vi "AudioTest.Plot, Normalize Freq Response Plot.vi"(6 "Average(F), Center_Min_Max(T)":bool, 8 "F End":dbl=20000.0, 9 "F Start":dbl=500.0, 11 "Data In":T1) -> (1 "Avg Level":T2 {"Status" items=["LOG", "PASS", "FAIL", "ERROR"]}, 3 "Data Out":T1)   [LabVIEW 2018]
uses:
  TypeDefs/AudioTest.Result Plot Data.ctl
  Common/Utils/Results/Result.Numeric.ctl
  Common/Utils/Results/Result.Limit Type.ctl
  Common/Utils/Results/Result.Measurement and Attribute Item Status.ctl
panel:
  in  "Limits In":T1[](array[typedef])
  out "XY Graph Out":cluster{"X":dbl[], dbl[]}(graph)
  out "XY Graph":cluster{"X":dbl[], "Y":dbl[]}(graph)
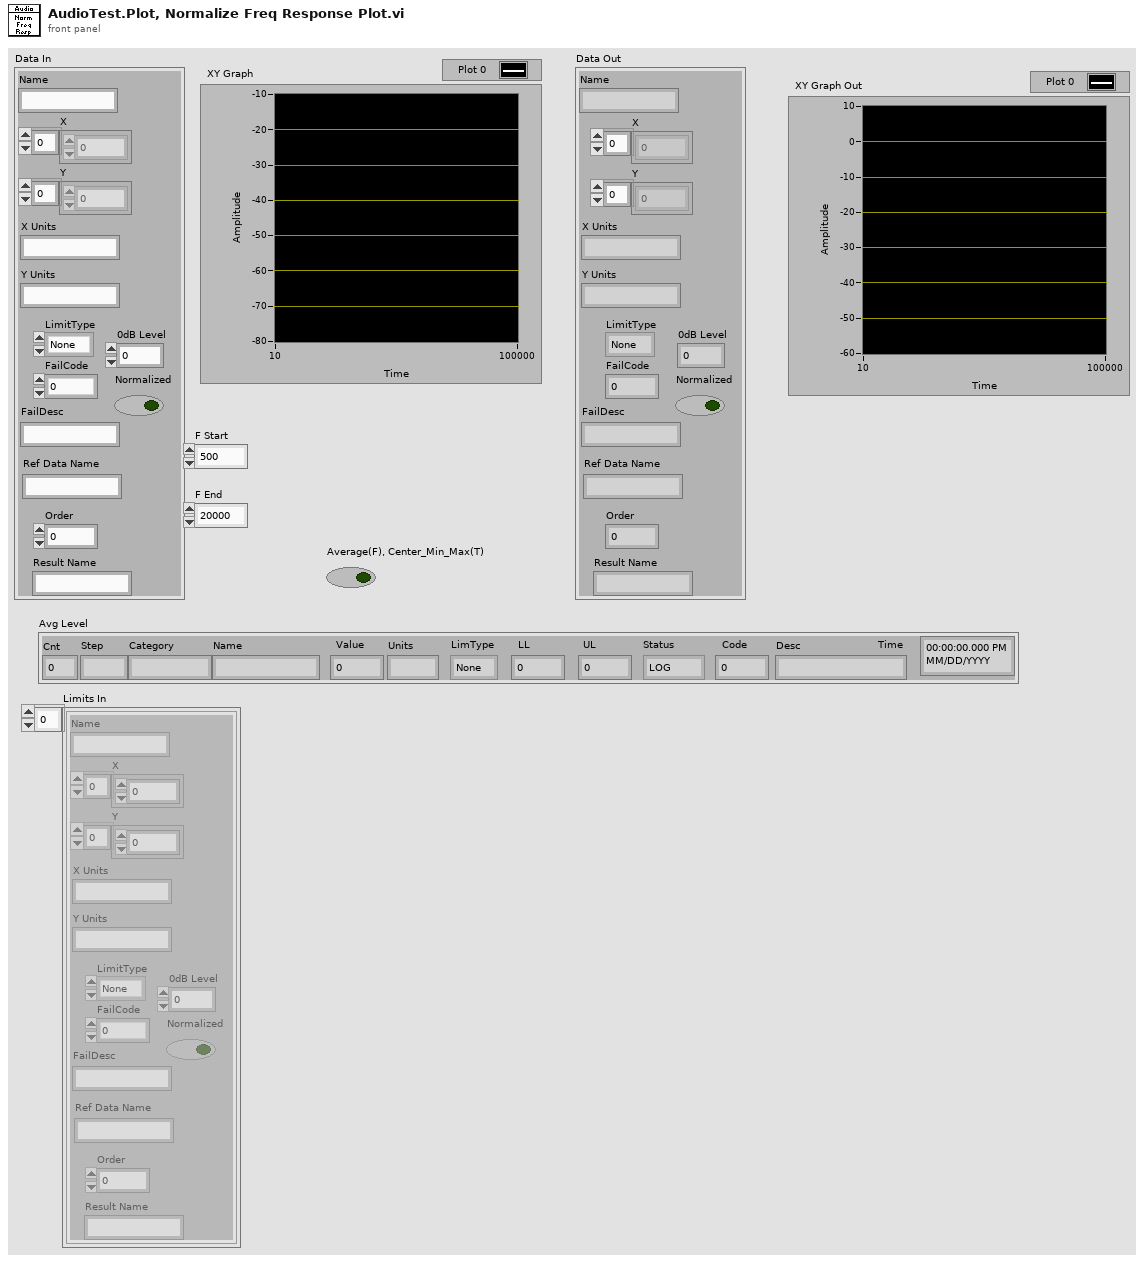
[diagram p1: front panel]
types:
  T1 = typedef "AudioTest.Result Plot Data.ctl" = cluster{"Order":i32, "Name":string, "X":dbl[], "Y":dbl[], "X Units":string, "Y Units":string, "LimitType":enum16{"None", "LL", "UL"}, "FailCode":i32, "FailDesc":string, "Ref Data Name":string, "Result Name":string, "0dB Level":dbl, "Normalized":bool}
  T2 = typedef "Result.Numeric.ctl" = cluster{"Cnt":i32, "Step":string, "Category":string, "Name":string, "Value":dbl, "Units":string, "LimType":T3, "LL":dbl, "UL":dbl, "Status":T4, "Code":i32, "Desc":string, "Time":timestamp}
  T3 = typedef "Result.Limit Type.ctl" = enum16{"None", "EQ", "NE", "GT", "LT", "GE", "LE", "GTLT", "GELE", "GELT", "GTLE", "LTGT", "LEGE", "LEGT", "LTGE", "Contains", "NotContains"}
  T4 = typedef "Result.Measurement and Attribute Item Status.ctl" = i32
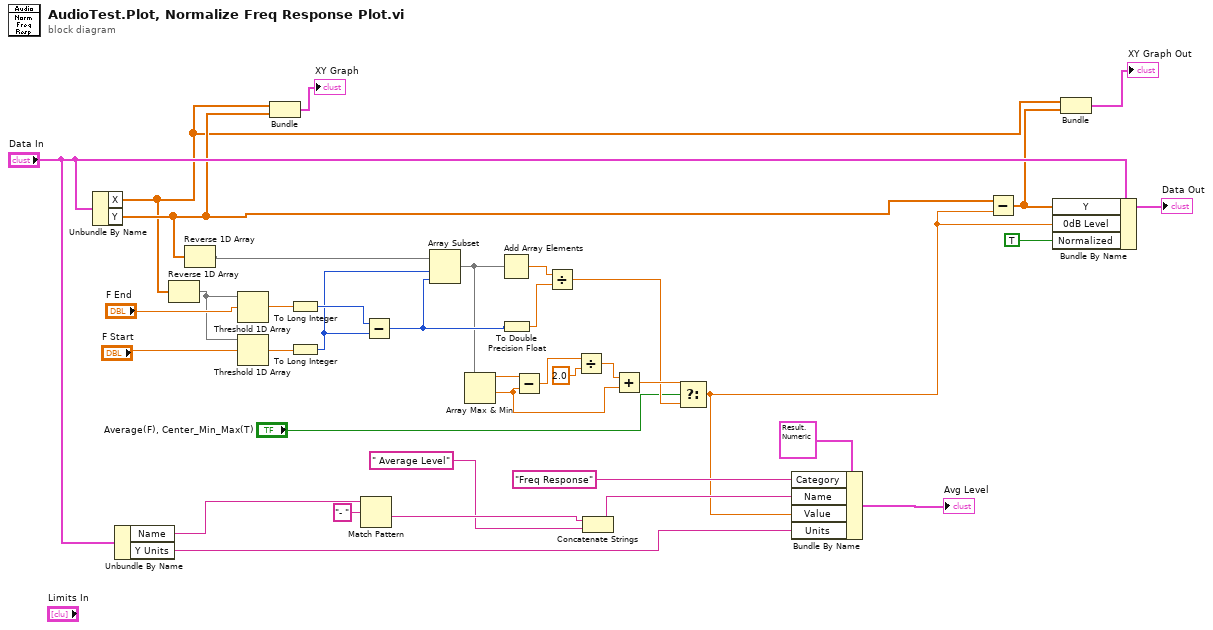
[diagram p0: block diagram]
diagram:
  n1 = Unbundle By Name("Data In") -> ("X"=w17:dbl[], "Y"=w19:dbl[])
  n2 = Unbundle By Name("Data In") -> ("Name"=w15:string, "Y Units"=w26:string)
  n3 = Reverse 1D Array(array=w17) -> (reversed array=w16:dbl[])
  n4 = Reverse 1D Array(array=w19) -> (reversed array=w18:dbl[])
  n5 = Threshold 1D Array(2:"F End", 3:w16) -> (0:w37:dbl)  [unwired: 1 in]
  n6 = Threshold 1D Array(2:"F Start", 3:w16) -> (0:w36:dbl)  [unwired: 1 in]
  n7 = Bundle("X"=w17, "Y"=w19) -> (→"XY Graph":cluster{"X":dbl[], "Y":dbl[]})  [unwired: 1 in]
  n8 = To Long Integer(number=w37) -> (32bit integer=w34:i32)
  n9 = To Long Integer(number=w36) -> (32bit integer=w33:i32)
  n10 = Match Pattern(string=w15, regular expression="- ") -> (after substring=w13:string)  [unwired: 1 in, 3 out]
  n11 = Subtract(x=w34, y=w33) -> (x-y=w30:i32)
  n12 = Array Subset(array=w18, index=w33, length=w30) -> (w11:dbl[])
  n13 = Array Max & Min(array=w11) -> (max value=w10:dbl, min value=w3:dbl)  [unwired: 2 out]
  n14 = Add Array Elements(numeric array=w11) -> (sum=w32:dbl)
  n15 = To Double Precision Float(number=w30) -> (double precision float=w31:dbl)
  n16 = Subtract(x=w10, y=w3) -> (x-y=w6:dbl)
  n17 = Divide(x=w32, y=w31) -> (x/y=w8:dbl)
  n18 = Divide(x=w6, y=2.0) -> (x/y=w4:dbl)
  n19 = Concatenate Strings(w13, " Average Level" ("Category")) -> (w27:string)
  n20 = Add(x=w4, y=w3) -> (x+y=w9:dbl)
  n21 = Select(t=w9, s="Average(F), Center_Min_Max(T)", f=w8) -> (s? t:f=w1:dbl)
  n22 = Bundle By Name(cluster=T2 {"Cnt"=0, "Step"="", "Category"="", "Name"="", "Value"=0.0, "Units"="", "LimType"=enum."None", "LL"=0.0, "UL"=0.0, "Status"=0, "Code"=0, "Desc"="", "Time"=timestamp(0 s since 1904-01-01)} ("Measurement"), "Category"="Freq Response", "Name"=w27, "Value"=w1, "Units"=w26) -> (→"Avg Level":T2)
  n23 = Subtract(x=w19, y=w1) -> (x-y=w22:dbl[])
  n24 = Bundle By Name(cluster="Data In", "Y"=w22, "0dB Level"=w1, "Normalized"=TRUE) -> (→"Data Out":T1)
  n25 = Bundle("X"=w17, w22) -> (→"XY Graph Out":cluster{"X":dbl[], dbl[]})  [unwired: 1 in]
